vi "Send Update Parameters.vi"(7 "Message Priority (Normal)":T3=enum."Normal", 8 "error in (no error)":errorcluster, 10 "Signal Parameters":T1 {"Amplitude" format="%#_2g V"; "Frequency" format="%d Hz"}, 11 "Message Enqueuer":refnum<class "Message Enqueuer.lvclass">) -> (0 "error out":errorcluster, 3 "Message Enqueuer out":refnum<class "Message Enqueuer.lvclass">)   [LabVIEW 2020, in "Function Generator Actor.lvlib" / "Update Parameters Msg.lvclass"]
doc: "This VI sends the message to an actor."
uses:
  Update Parameters Msg.lvclass
  <vilib>/ActorFramework/Message Enqueuer/Message Enqueuer.lvclass
  <vilib>/ActorFramework/Message Enqueuer/Message Priority.ctl
  Controls/SignalParamTD.ctl
  Controls/SignalShapeTD.ctl
  C:/Program Files (x86)/National Instruments/LabVIEW 2020/vi.lib/ActorFramework/Message/Message.lvclass
  Update Parameters Msg.lvclass/Update Parameters Msg.ctl
  <vilib>/ActorFramework/Message Enqueuer/Message Enqueuer.lvclass/Message Enqueuer.ctl
  <vilib>/ActorFramework/Message Priority Queue/Priority Enqueue.vi
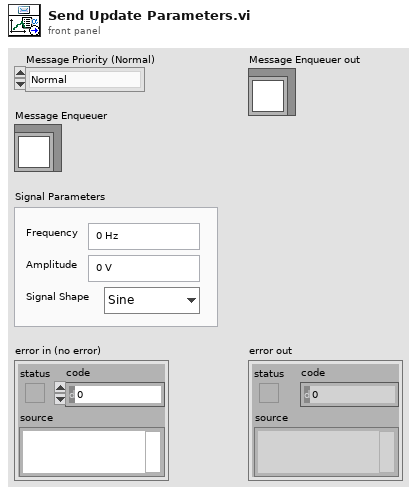
[diagram p1: front panel]
types:
  T1 = typedef "SignalParamTD.ctl" = cluster{"Frequency":u32, "Amplitude":dbl, "Signal Shape":T2}
  T2 = typedef "SignalShapeTD.ctl" = enum16{"Sine", "Square", "Triangle"}
  T3 = typedef "Actor Framework.lvlib/Message Enqueuer.lvclass/Message Priority.ctl" = enum16{"Low", "Normal", "High"}
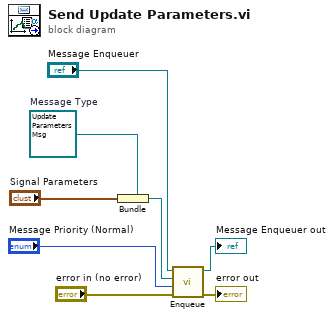
[diagram p0: block diagram]
diagram:
  w5 = refnum<class "Update Parameters Msg.lvclass"> refnum  # Message Type
  n1 = Bundle(cluster=w5, "Signal Parameters") -> (w4:refnum<class "Update Parameters Msg.lvclass">)
  n2 = call <vilib>:"Enqueue.vi"("error in (no error)"="error in (no error)", "Message Priority (Normal)"="Message Priority (Normal)", "Message"=w4, "Message Enqueuer in"="Message Enqueuer") -> ("error out"=→"error out":errorcluster, "Message Enqueuer out"=→"Message Enqueuer out":refnum<class "Message Enqueuer.lvclass">)  [unwired: 6 in]
